vi "Display Unicode Strings in Ring Control.vi"() -> ()   [LabVIEW 2020]
panel:
  in  "Unicode":bool
  in  "Ring":u16(ring) items=["?@825B", "<8@", "ª0×0·0ç0ó0C"]
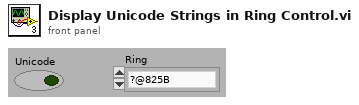
[diagram p1: front panel]
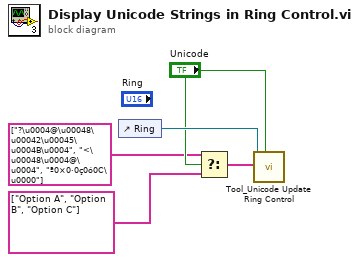
[diagram p0: block diagram]
diagram:
  n1 = control-ref of="Ring"() -> (w5:refnum<vi>)
  n2 = Select(t=string[] ["?\u0004@\u00048\u00042\u00045\u0004B\u0004", "<\u00048\u0004@\u0004", "ª0×0·0ç0ó0C\u0000"], s="Unicode", f=string[] ["Option A", "Option B", "Option C"]) -> (s? t:f=w1:string[])
  n3 = call "Tool_Unicode Update Ring Control.vi"("Interpret as Unicode (T)"="Unicode", "Strings"=w1, "Ring Control Ref"=w5) -> ()  [unwired: 6 in, 1 out]
